vi "Read State.vi"(8 "error in (no error)":errorcluster, 11 "TwinCAT ADS in":refnum<class "TwinCAT ADS.lvclass">) -> (0 "error out":errorcluster, 1 "State Information":T1 {"ADS State" items=["Invalid", "Idle", "Reset", "Init", "Start", "Run", "Stop", "SaveConfig", "LoadConfig", "PowerFailure", "PowerGood", "Error", "Shutdown", "Suspend", "Resume", "Config", "Reconfig", "Stopping, Maxstates", "Incompatible", "Exception"]}, 3 "TwinCAT ADS out":refnum<class "TwinCAT ADS.lvclass">)   [LabVIEW 2018, in "TwinCAT ADS.lvclass"]
uses:
  TwinCAT ADS.lvclass
  Controls/State Information.ctl
  TwinCAT.Ads
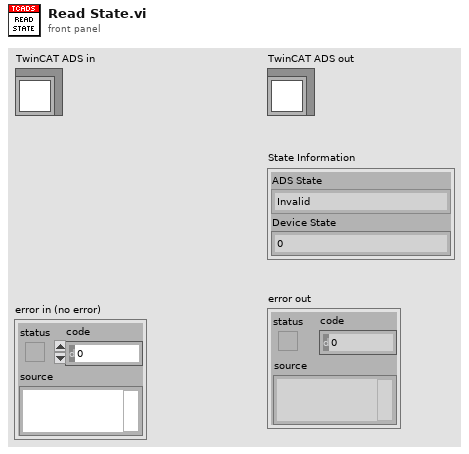
[diagram p1: front panel]
types:
  T1 = typedef "TwinCAT ADS.lvclass/State Information.ctl" = cluster{"ADS State":i16, "Device State":i16}
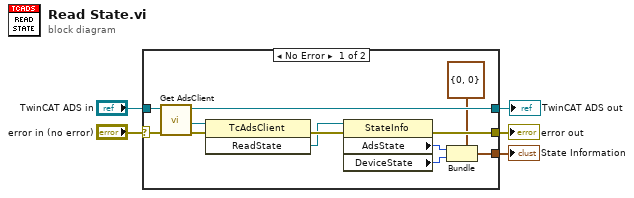
[diagram p0: block diagram]
diagram:
  n1 = case shown="No Error" "error in (no error)" {
    selector: "error in (no error)" -> [w11 w19]
    tunnel: [w15 w19] -> w4
    tunnel: [w7 w18] -> w2
    tunnel: "TwinCAT ADS in" -> [w8 w18]
    tunnel: [w12 _] -> w1
    frame No Error {
      n2 = call-dynamic "Get AdsClient.vi"("error in (no error)"=w11, "TwinCAT ADS in"=w8) -> ("error out"=w10:errorcluster, ".NET TcAdsClient refnum"=w9:refnum<k24>, "TwinCAT ADS out"=w7:refnum<class "TwinCAT ADS.lvclass">)  [unwired: 7 in]
      n3 = invoke class="TcAdsClient" method="ReadState"(reference=w9, error in=w10) -> (error out=w17:errorcluster, "ReadState"=w16:refnum<k24>)  [unwired: 1 in, 1 out]
      n4 = property class="StateInfo"(reference=w16, error in=w17) -> (error out=w15:errorcluster, "AdsState"=w14:i16, "DeviceState"=w13:i16)  [unwired: 1 out]
      n5 = Bundle(cluster=T1 {"ADS State"=0, "Device State"=0} ("State Information"), "ADS State"=w14, "Device State"=w13) -> (w12:T1)
    }
    frame Error {
    }
  }
  "error out" <- w4
  "TwinCAT ADS out" <- w2
  "State Information" <- w1
